vi "Panel RefGlb.vi"() -> ()   [LabVIEW 2019]
panel:
  in  "Process load":bool
  in  "IO load":bool
  in  "Virbration load":bool
  in  "vision load":bool
  out "PanelRef":refnum<vi>[](array[refnum])
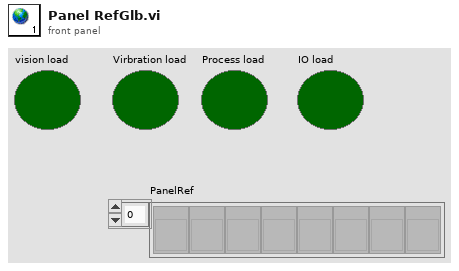
[diagram p1: front panel]
diagram:
